vi "Get Baratron Voltage.vi"(8 "error in (no error)":errorcluster, 10 "Baratron Voltage":waveform(dbl)[](array[waveform]), 11 "Baratron in":refnum<class "Baratron.lvclass">) -> (0 "error out":errorcluster, 3 "Baratron out":refnum<class "Baratron.lvclass">)   [LabVIEW 2021, in "Baratron.lvlib" / "Baratron.lvclass"]
uses:
  Baratron.lvclass
  Baratron.lvclass/Baratron.ctl
  <vilib>/ActorFramework/Actor/Actor.lvclass
  Baratron Pressure/Baratron Pressure Messages/Baratron Pressure Msg/Baratron Pressure Msg.lvclass
  <vilib>/NathanCo/Analog-Tasks/Analog Input/Analog Input/Analog Input/Analog Input.lvclass
  C:/Program Files/National Instruments/LabVIEW 2021/vi.lib/MGI/Panel Manager/Panel Actor/Panel Actor/Panel Actor.lvclass
  C:/Program Files/National Instruments/LabVIEW 2021/vi.lib/ActorFramework/Actor/Actor.lvclass
  C:/git/Pressure-Gauges/Files-to-be-organized/Baratron/Baratron/Baratron.lvclass
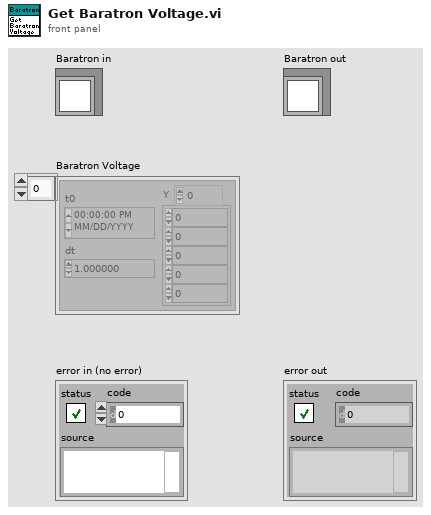
[diagram p1: front panel]
types:
  T1 = typedef "Baratron.lvlib/Baratron.lvclass/Status Range.ctl" = enum16{"Above Range", "Below Range", "Within Range"}
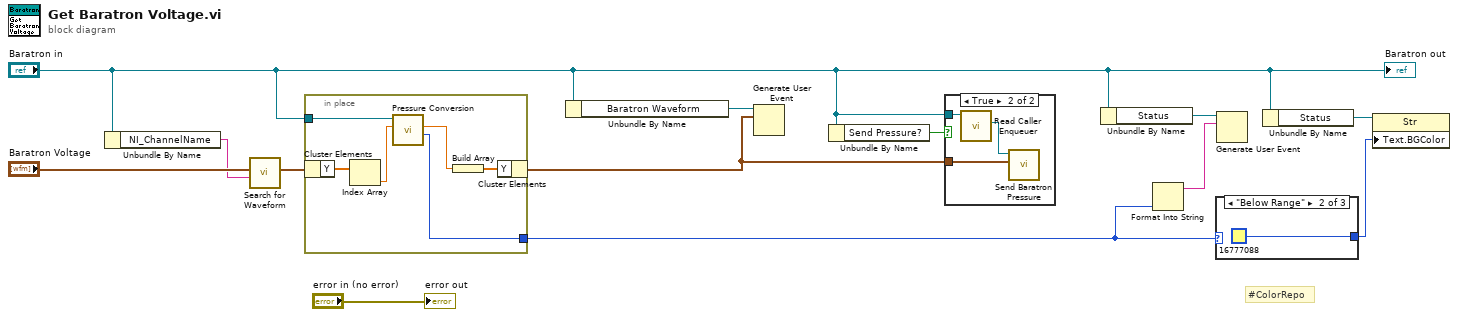
[diagram p0: block diagram]
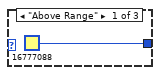
[diagram p3: hidden frame]
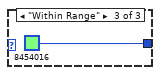
[diagram p4: hidden frame]
diagram:
  # "#ColorRepo"
  n1 = Unbundle By Name("Baratron in") -> ("NI_ChannelName"=w2:string)
  n2 = call <vilib>:"Search for Waveform.vi"("NI_ChannelName"=w2, "Waveforms"="Baratron Voltage") -> ("Waveform"=w1:waveform(dbl))  [unwired: 8 in, 1 out]
  n3 = in-place {
    in-place-border: [w16] -> w8
    in-place-border: "Baratron in" -> [w15]
    n4 = in-place-cluster #1(w1) -> ("Y"=w17:dbl[])
    n5 = Index Array(array=w17) -> (element=w18:dbl)  [unwired: 1 in]
    n6 = call "Pressure Conversion.vi"("Voltage"=w18, "Baratron in"=w15) -> ("Status Range"=w16:T1, "Pressure"=w14:dbl)  [unwired: 8 in]
    n7 = Build Array(w14) -> (w19:dbl[])
    n8 = in-place-cluster #1("Y"=w19) -> (w5:waveform(dbl))
  }
  n9 = Unbundle By Name("Baratron in") -> ("Baratron Waveform"=w12:refnum<user-event>)
  n10 = Generate User Event(user event=w12, event data cluster=w5) -> ()  [unwired: 2 in, 2 out]
  n11 = Unbundle By Name("Baratron in") -> ("Send Pressure?"=w6:bool)
  n12 = case shown="True" w6 {
    tunnel: "Baratron in" -> [_ w21]
    tunnel: w5 -> [_ w20]
    frame False {
    }
    frame True {
      n13 = call <vilib>:"Read Caller Enqueuer.vi"("Actor"=w21) -> ("Caller Enqueuer"=w22:refnum<class "Message Enqueuer.lvclass">)  [unwired: 10 in]
      n14 = call "Send Baratron Pressure.vi"("Baratron Pressure"=w20, "Message Enqueuer"=w22) -> ()  [unwired: 8 in, 2 out]
    }
  }
  n15 = Unbundle By Name("Baratron in") -> ("Status"=w10:refnum<user-event>)
  n16 = Format Into String(w8) -> (resulting string=w9:string)  [unwired: 3 in, 1 out]
  n17 = case shown="\"Below Range\"" w8 {
    tunnel: [u32 16777088 ("Text.Colors:BG Color") u32 16777088 ("Text.Colors:BG Color") u32 8454016 ("Text.Colors:BG Color")] -> w7
    frame "Above Range" {
    }
    frame "Below Range" {
    }
    frame "Within Range" {
    }
  }
  n18 = Generate User Event(user event=w10, event data cluster=w9) -> ()  [unwired: 2 in, 2 out]
  n19 = Unbundle By Name("Baratron in") -> ("Status"=w11:refnum<vi>)
  n20 = property class="Str"(reference=w11, "Text.BGColor"=w7) -> ()  [unwired: 1 in, 2 out]
  "error out" <- "error in (no error)"
  "Baratron out" <- "Baratron in"
